vi "gaussian random walk.vi"() -> ()   [LabVIEW 2014]
uses:
  <vilib>/userdefined/High Color/IMAQdx.ctl
  <vilib>/Utility/file.llb/Write To Spreadsheet File (DBL).vi
  <vilib>/vision/driver/NI_Vision_Acquisition_Software.lvlib
panel:
  in  "Start Recording":bool
  in  "Max Voltage":dbl
  in  "Min Voltage":dbl
  in  "Frames":i32
  in  "Sigma":dbl
  in  "Initial Voltage":dbl
  out "Error":string
  out "Save Directory":path
  out "Buffer Number Out":u32
  out "Image":T1(plugin-control)
  in  "stop":bool
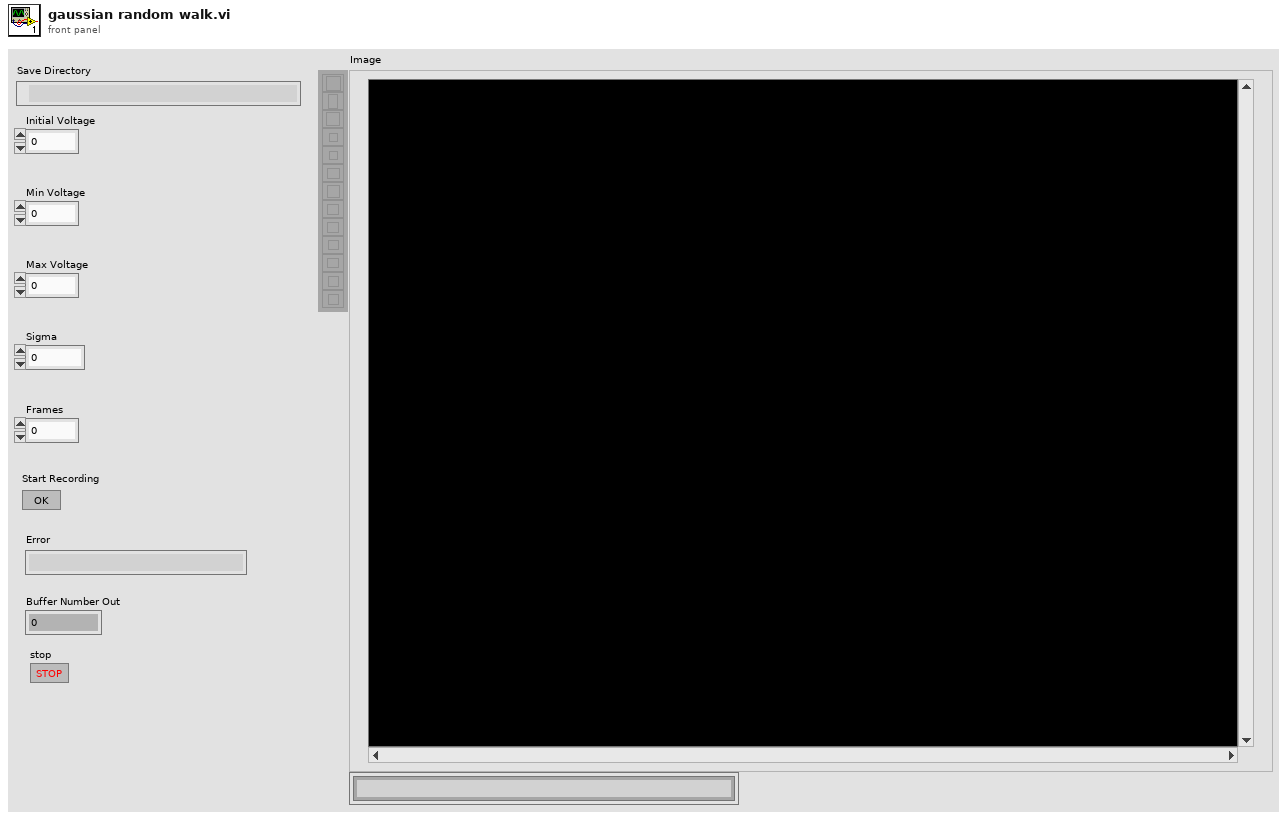
[diagram p1: front panel]
types:
  T1 = typedef "IMAQ Image.ctl" = refnum<image>
  T2 = typedef "IMAQdx.ctl" = refnum<k21>
  T3 = cluster{"Rows Per Strip":i32, "Photometric":i32, "Compression Type":i32}
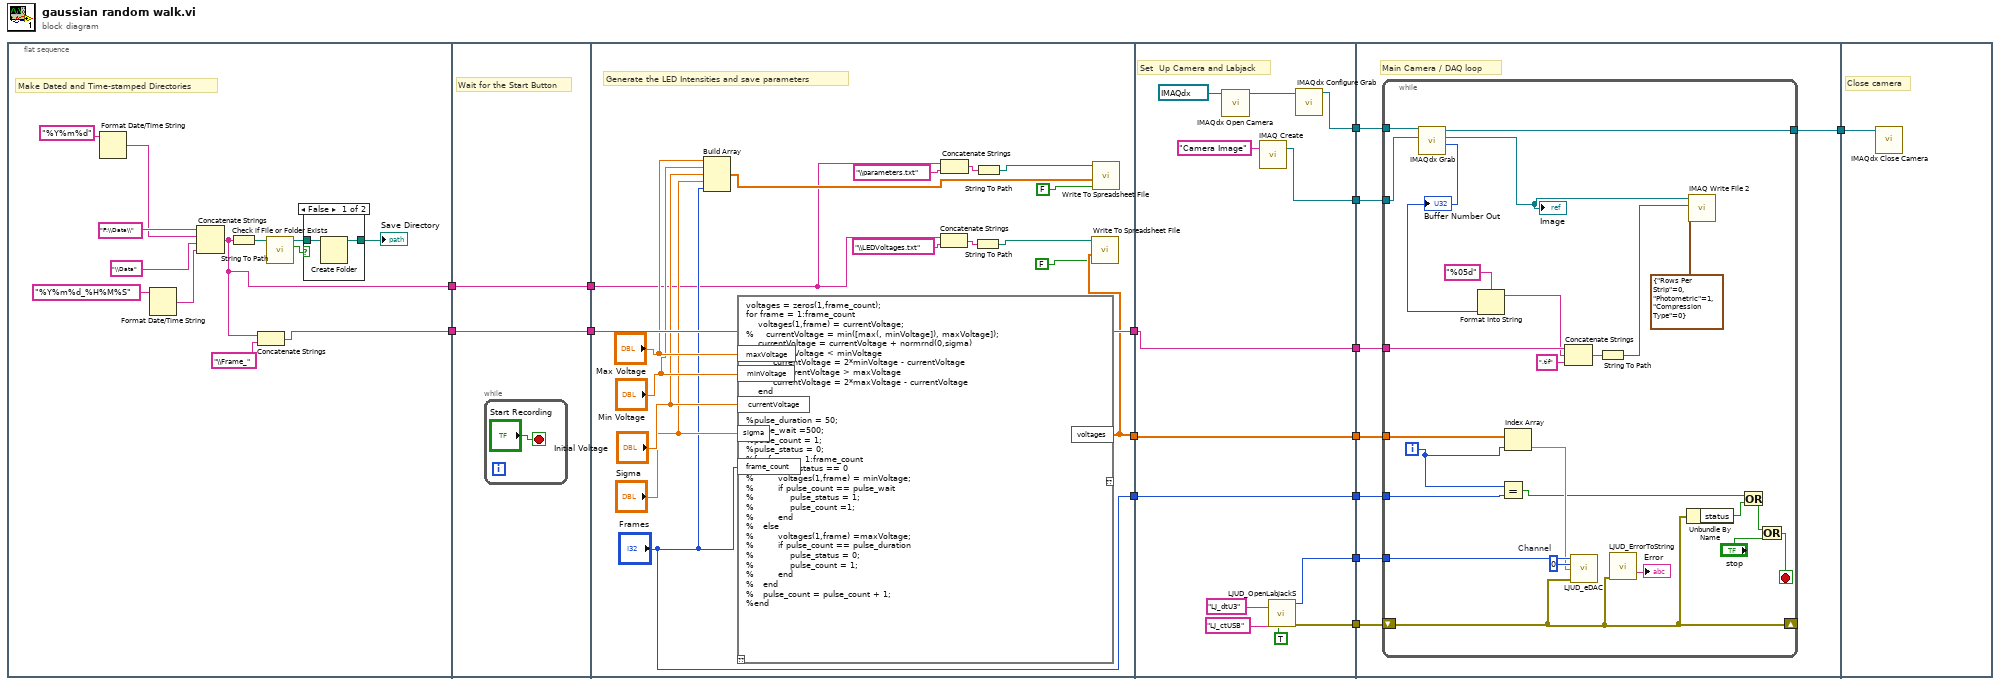
[diagram p0: block diagram]
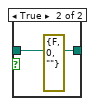
[diagram p2: hidden frame]
diagram:
  n1 = flat-sequence {
    tunnel: [w18] -> w4
    tunnel: [w16] -> w2
    tunnel: w4 -> [w33]
    tunnel: [w33] -> w3
    tunnel: w2 -> [w32]
    tunnel: [w32] -> w1
    tunnel: w3 -> [w49]
    tunnel: [w49] -> w9
    tunnel: [w47] -> w7
    tunnel: ["Frames"] -> w6
    tunnel: w1 -> [w35]
    tunnel: w9 -> [w59]
    tunnel: [w61] -> w15
    tunnel: [w60] -> w14
    tunnel: [w59] -> w13
    tunnel: [w55] -> w11
    tunnel: [w54] -> w10
    tunnel: [w53] -> w8
    tunnel: w7 -> [w53]
    tunnel: w6 -> [w52]
    tunnel: [w52] -> w5
    tunnel: w15 -> [w72]
    tunnel: w14 -> [w71]
    tunnel: w13 -> [w70]
    tunnel: [w69] -> w12
    tunnel: w11 -> [w68]
    tunnel: w10 -> [w67]
    tunnel: w8 -> [w66]
    tunnel: w5 -> [w65]
    tunnel: w12 -> [w98]
    frame #0 {
      # "Make Dated and Time-stamped Directories"
      n2 = Format Date/Time String(time format string (%c)="%Y%m%d") -> (date/time string=w19:string)  [unwired: 2 in]
      n3 = Format Date/Time String(time format string (%c)="%Y%m%d_%H%M%S") -> (date/time string=w23:string)  [unwired: 2 in]
      n4 = Concatenate Strings("F:\\Data\\", w19, "\\Data", w23) -> (w16:string)
      n5 = String To Path(string=w16) -> (path=w22:path)
      n6 = Concatenate Strings(w16, "\\Frame_") -> (w18:string)
      n7 = call <vilib>:"Check if File or Folder Exists.vi"("path"=w22) -> ("file or folder exists?"=w27:bool, "dup path"=w26:path)  [unwired: 8 in, 1 out]
      n8 = case shown="False" w27 {
        tunnel: [w29 w31] -> w21
        tunnel: w26 -> [w30 w31]
        frame False {
          n9 = Create Folder(path (use dialog)=w30) -> (created path=w29:path)  [unwired: 2 in, 2 out]
        }
        frame True {
          (unwired) errorcluster {"status"=FALSE, "code"=0, "source"=""} ("error out")
        }
      }
      "Save Directory" <- w21
    }
    frame #1 {
      # "Wait for the Start Button"
      n10 = while {
        stop <- "Start Recording" stop-if-true
      }
    }
    frame #2 {
      # "Generate the LED Intensities and save parameters"
      n11 = Build Array("Max Voltage", "Min Voltage", "Initial Voltage", "Sigma", "Frames") -> (w36:dbl[])
      n12 = script code="voltages = zeros(1,frame_count);\nfor frame = 1:frame_count\n    voltages(1,frame) = currentVoltage;\n%    currentVoltage = min([max(, minVoltage]), maxVoltage]);\n    currentVoltage = currentVoltage + normrnd(0,sigma)\n    if currentVoltage < minVoltage\n         currentVoltage = 2*minVoltage - currentVoltage\n    elseif currentVoltage > maxVoltage\n         currentVoltage = 2*maxVoltage - currentVoltage\n    end\nend\n\n%pulse_duration = 50;\n%pulse_wait =500;\n%pulse_count = 1;\n%pulse_status = 0;\n%for frame = 1:frame_count\n%    if pulse_status == 0\n%        voltages(1,frame) = minVoltage;\n%        if pulse_count == pulse_wait\n%            pulse_status = 1;\n%            pulse_count =1;\n%        end\n%   else\n%        voltages(1,frame) =maxVoltage;\n%        if pulse_count == pulse_duration\n%            pulse_status = 0;\n%            pulse_count = 1;\n%        end\n%   end\n%   pulse_count = pulse_count + 1;\n%end"("currentVoltage"="Initial Voltage", "frame_count"="Frames", "sigma"="Sigma", "minVoltage"="Min Voltage", "maxVoltage"="Max Voltage") -> ("voltages"=w47:dbl[])  [unwired: 1 in, 1 out]
      n13 = Concatenate Strings(w35, "\\LEDVoltages.txt") -> (w51:string)
      n14 = Concatenate Strings(w35, "\\parameters.txt") -> (w40:string)
      n15 = String To Path(string=w51) -> (path=w50:path)
      n16 = String To Path(string=w40) -> (path=w39:path)
      n17 = call-poly <vilib>:"Write To Spreadsheet File.vi"("append to file? (new file:F)"=FALSE, "1D data"=w47, "file path (dialog if empty)"=w50) -> ()  [unwired: 5 in, 1 out]
      n18 = call-poly <vilib>:"Write To Spreadsheet File.vi"("append to file? (new file:F)"=FALSE, "1D data"=w36, "file path (dialog if empty)"=w39) -> ()  [unwired: 5 in, 1 out]
    }
    frame #3 {
      # "Set  Up Camera and Labjack"
      n19 = call <vilib>:"IMAQdx Open Camera.vi"("Session In"=T2 "cam0") -> ("Session Out"=w63:T2)  [unwired: 9 in, 1 out]
      n20 = call "IMAQ Create"("Image Name"="Camera Image") -> ("New Image"=w60:T1)  [unwired: 4 in, 1 out]
      n21 = call "LJUD_OpenLabJackS.vi"("FirstFound"=TRUE, "ConnectionType"="LJ_ctUSB", "DeviceType"="LJ_dtU3") -> ("error out"=w54:errorcluster, "Handle"=w55:i32)  [unwired: 6 in, 1 out]
      n22 = call <vilib>:"IMAQdx Configure Grab.vi"("Session In"=w63) -> ("Session Out"=w61:T2)  [unwired: 9 in, 1 out]
    }
    frame #4 {
      # "Main Camera / DAQ loop"
      n23 = while {
        tunnel: w72 -> [w97]
        tunnel: [w96] -> w69
        tunnel: w71 -> [w95]
        tunnel: w70 -> [w93]
        tunnel: w68 -> [w85]
        shift-right: [w82] -> _
        shift-left: w67 -> [w82]
        tunnel: w66 -> [w74]
        tunnel: w65 -> [w73]
        i -> [w75]
        stop <- w84 stop-if-true
        w81 = 0  # Channel
        n24 = call <vilib>:"IMAQdx Grab.vi"("Image In"=w95, "Session In"=w97) -> ("Buffer Number Out"=w88:u32, "Image Out"=w94:T1, "Session Out"=w96:T2)  [unwired: 6 in, 1 out]
        "Image" <- w94
        "Buffer Number Out" <- w88
        n25 = Format Into String(format string="%05d" ("string"), w88) -> (resulting string=w87:string)  [unwired: 2 in, 1 out]
        n26 = Equal?(x=w75, y=w73) -> (x = y?=w77:bool)
        n27 = Index Array(array=w74, index=w75) -> (element=w79:dbl)
        n28 = Concatenate Strings(w93, w87, ".tif" ("string")) -> (w91:string)
        n29 = call "LJUD_eDAC.vi"("Handle In"=w85, "Channel"=w81, "Voltage"=w79, "error in"=w82) -> ()  [unwired: 10 in, 2 out]
        n30 = String To Path(string=w91) -> (path=w90:path)
        n31 = call "LJUD_ErrorToString.vi"("error in"=w82) -> ("String"=→"Error":string)  [unwired: 10 in]
        n32 = Unbundle By Name(w82) -> ("status"=w78:bool)
        n33 = call-poly "IMAQ Write File 2"("TIFF Options"=T3 {"Rows Per Strip"=0, "Photometric"=1, "Compression Type"=0}, "File Path"=w90, "Image"=w94) -> ()  [unwired: 7 in, 2 out]
        n34 = Or(x=w77, y=w78) -> (x .or. y?=w76:bool)
        n35 = Or(x=w76, y="stop") -> (x .or. y?=w84:bool)
      }
    }
    frame #5 {
      # "Close camera"
      n36 = call <vilib>:"IMAQdx Close Camera.vi"("Session In"=w98) -> ()  [unwired: 10 in, 1 out]
    }
  }
